vi "3458 Conf-trig.vi"(2 "error in":errorcluster, 5 "address string":string) -> (0 "error out":errorcluster, 1 "timeout ms (488.2 global)":i32=120000)   [LabVIEW 2014]
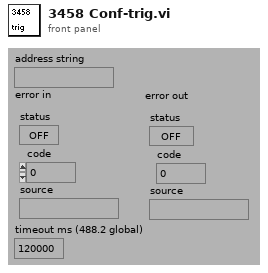
[diagram p1: front panel]
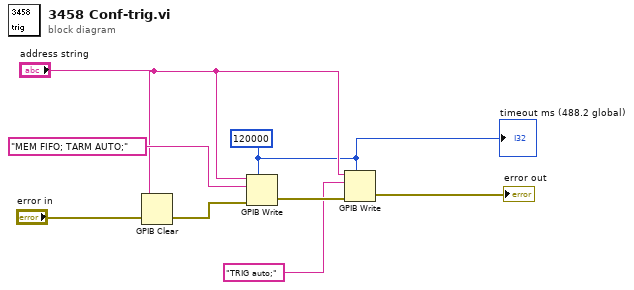
[diagram p0: block diagram]
diagram:
  w1 = 120000 ("timeout ms (488.2 global)")
  n1 = GPIB Clear(2:"error in", 3:"address string") -> (0:w6:errorcluster)  [unwired: 1 out]
  n2 = GPIB Write(0:"address string", 1:"MEM FIFO; TARM AUTO;", 3:w6, 4:w1) -> (6:w5:errorcluster)  [unwired: 1 in, 1 out]
  n3 = GPIB Write(0:"address string", 1:"TRIG auto;", 3:w5, 4:w1) -> (6:→"error out":errorcluster)  [unwired: 1 in, 1 out]
  "timeout ms (488.2 global)" <- w1
